vi "Launcher_Main.vi"   [LabVIEW 2020]
uses:
  #typedef_Launcher_States.ctl
  Controller/#typedef_ControllerQueue_States.ctl
types:
  T1 = typedef "#typedef_Launcher_States.ctl" = enum16{"ERROR_Default", "StartApp", "InitIntermoduleQueueComm", "InitModules", "Run", "CloseIntermoduleQueueComm", "CloseApp"}
  T2 = typedef "#typedef_ControllerQueue_States.ctl" = enum16{"ERROR_Default", "Obtain", "GetRef", "Enqueue", "EnqueueAtOpp", "GetStatus", "Flush", "Release"}
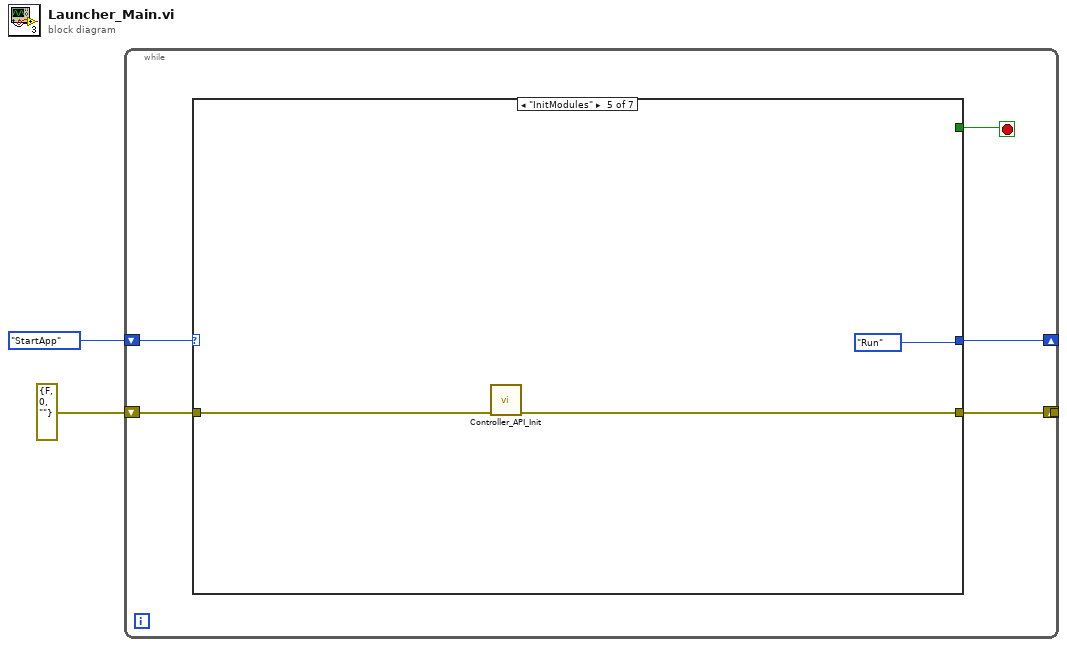
[diagram p0: block diagram]
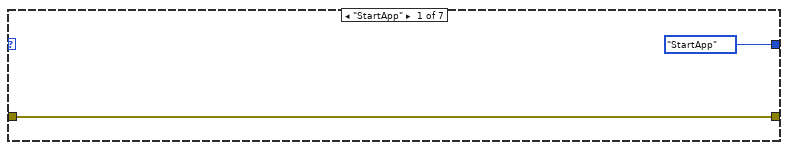
[diagram p2: hidden frame]
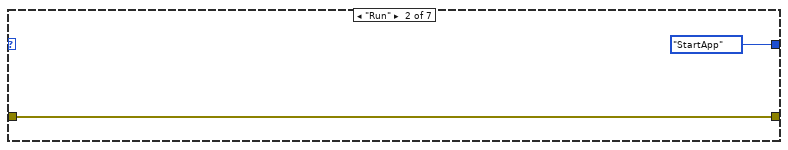
[diagram p3: hidden frame]
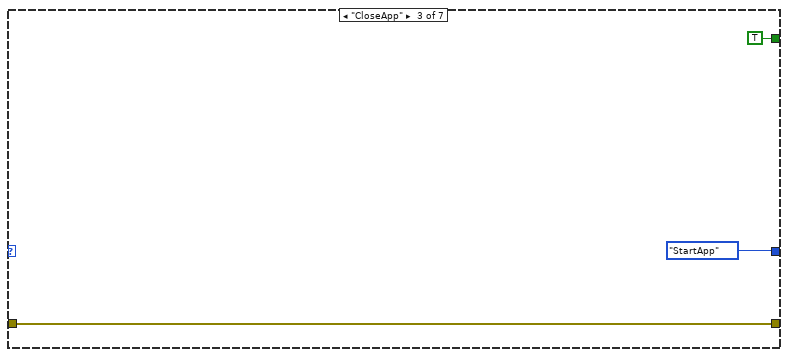
[diagram p4: hidden frame]
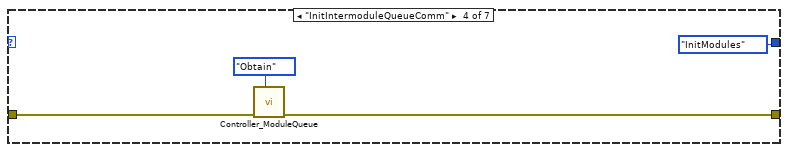
[diagram p5: hidden frame]
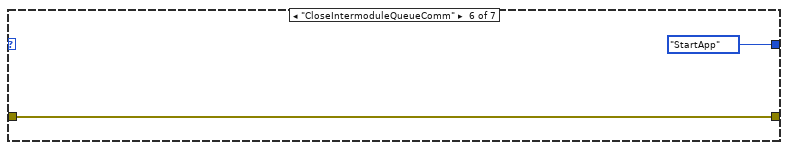
[diagram p6: hidden frame]
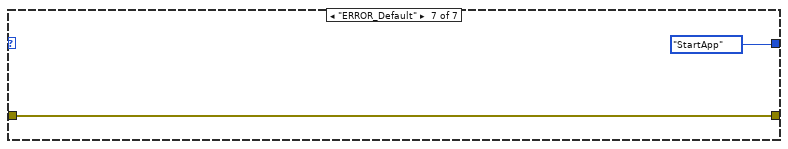
[diagram p7: hidden frame]
diagram:
  n1 = while {
    tunnel: [w5] -> _
    shift-right: _ -> [_]
    shift-left: errorcluster {"status"=FALSE, "code"=0, "source"=""} ("error in (no error)") -> [w6]
    shift-right: [w4] -> _
    shift-left: #typedef_Launcher_States."StartApp" -> [w7]
    stop <- w3 stop-if-true
    n2 = case shown="\"InitModules\"" w7 {
      tunnel: w6 -> [w8 w11 w12 w17 w20 w22 w24]
      tunnel: [w8 w11 w12 w15 w19 w22 w24] -> w5
      tunnel: [#typedef_Launcher_States."StartApp" #typedef_Launcher_States."StartApp" #typedef_Launcher_States."StartApp" #typedef_Launcher_States."InitModules" #typedef_Launcher_States."Run" #typedef_Launcher_States."StartApp" #typedef_Launcher_States."StartApp"] -> w4
      tunnel: [_ _ TRUE _ _ _ _] -> w3
      frame "StartApp" {
      }
      frame "Run" {
      }
      frame "CloseApp" {
      }
      frame "InitIntermoduleQueueComm" {
        n3 = call "Controller_ModuleQueue.vi"("Enum"=#typedef_ControllerQueue_States."Obtain", "error in (no error)"=w17) -> ("error out"=w15:errorcluster)  [unwired: 6 in, 3 out]
      }
      frame "InitModules" {
        n4 = call "Controller_API_Init.vi"("error in (no error)"=w20) -> ("error out"=w19:errorcluster)  [unwired: 10 in]
      }
      frame "CloseIntermoduleQueueComm" {
      }
      frame "ERROR_Default" {
      }
    }
  }
